vi "Do Something.vi"(8 "error in (no error)":errorcluster, 10 "Lithography Data":T2(array[cluster]), 11 "Instrument.AFM_DLog in":refnum<class "Instrument.AFM_DLog.lvclass">) -> (0 "error out":errorcluster, 3 "Instrument.AFM_DLog out":refnum<class "Instrument.AFM_DLog.lvclass">)   [LabVIEW 2019, in "Instrument.AFM_DLog.lvclass"]
uses:
  Instrument.AFM_DLog.lvclass
  <userlib>/LevyLab/Relay Box/Typedefs/Resistor--enum.ctl
  <userlib>/LevyLab/Relay Box/Relay-Box.lvclass
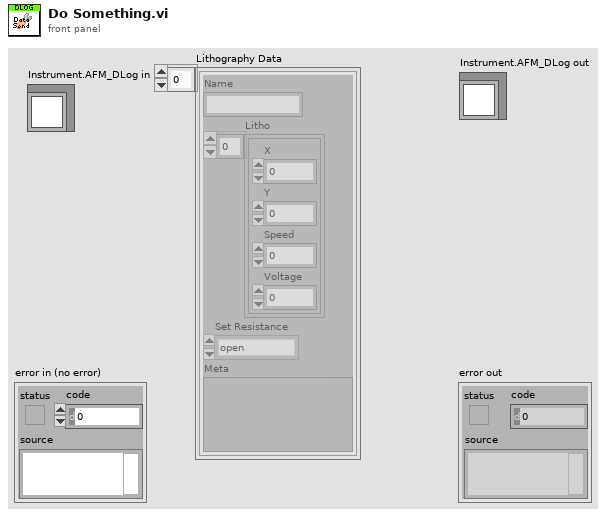
[diagram p1: front panel]
types:
  T1 = typedef "Relay-Box.lvclass/Resistor--enum.ctl" = enum16{"open", "discharge tip", "0 ohms", "100k ohm", "10M ohm", "1G ohm"}
  T2 = cluster{"Name":string, "Litho":cluster{"X":dbl, "Y":dbl, "Speed":dbl, "Voltage":dbl}[], "Set Resistance":T1, "Meta":variant}[]
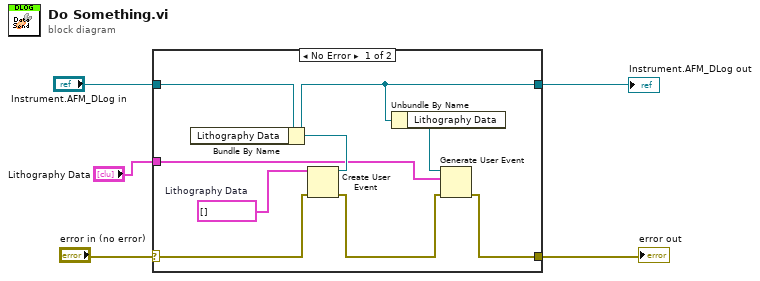
[diagram p0: block diagram]
diagram:
  n1 = case shown="No Error" "error in (no error)" {
    selector: "error in (no error)" -> [w14 w15]
    tunnel: [w7 w15] -> w3
    tunnel: [w6 w16] -> w5
    tunnel: "Instrument.AFM_DLog in" -> [w12 w16]
    tunnel: "Lithography Data" -> [w10 _]
    frame No Error {
      w13 = T2 []  # Lithography Data
      n2 = Create User Event(user event datatype=w13, error in=w14) -> (user event=w11:refnum<user-event>, error out=w8:errorcluster)
      n3 = Bundle By Name(cluster=w12, "Lithography Data"=w11) -> (w6:refnum<class "Instrument.AFM_DLog.lvclass">)
      n4 = Unbundle By Name(w6) -> ("Lithography Data"=w9:refnum<user-event>)
      n5 = Generate User Event(user event=w9, event data cluster=w10, error in=w8) -> (error out=w7:errorcluster)  [unwired: 1 in, 1 out]
    }
    frame Error {
    }
  }
  "error out" <- w3
  "Instrument.AFM_DLog out" <- w5
